vi "estimate_F_O.vi"(6 "lolo":dbl=10.0, 7 "hihi":dbl=100.0, 10 "F_O_now":dbl=1000.0, 11 "change":dbl) -> (2 "F_O_new":dbl)   [LabVIEW 2019]
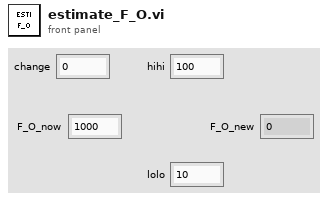
[diagram p1: front panel]
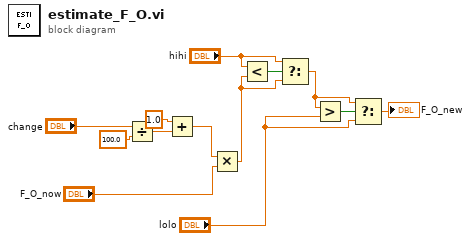
[diagram p0: block diagram]
diagram:
  n1 = Divide(x="change", y=100.0) -> (x/y=w10:dbl)
  n2 = Add(x=1.0, y=w10) -> (x+y=w8:dbl)
  n3 = Multiply(x=w8, y="F_O_now") -> (x*y=w6:dbl)
  n4 = Less?(x="hihi", y=w6) -> (x < y?=w7:bool)
  n5 = Select(t="hihi", s=w7, f=w6) -> (s? t:f=w2:dbl)
  n6 = Greater?(x=w2, y="lolo") -> (0:w4:bool)
  n7 = Select(t=w2, s=w4, f="lolo") -> (s? t:f=→"F_O_new":dbl)
